vi "Cartesian To Complex - R,RM.vi"(1 "Real Matrix I":T1, 2 "Real Scalar r":dbl) -> (0 "r + Ii":T2)   [LabVIEW 2017, in "NI_Matrix.lvlib"]
doc: "Creates a complex number from two values in rectangular notation."
uses:
  NI_Matrix.lvlib
  ComplexMatrix.ctl
  RealMatrix.ctl
  Array To Matrix - CA2.vi
  Matrix To Array - RM.vi
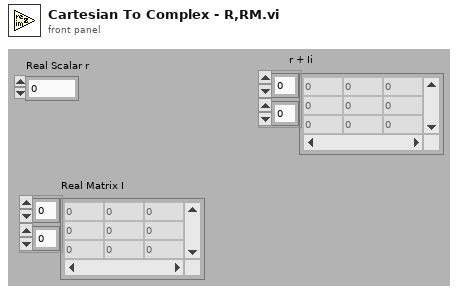
[diagram p1: front panel]
types:
  T1 = typedef "NI_Matrix.lvlib/RealMatrix.ctl" = dbl[][]
  T2 = typedef "NI_Matrix.lvlib/ComplexMatrix.ctl" = cdb[][]
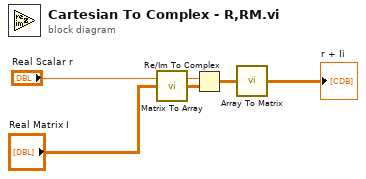
[diagram p0: block diagram]
diagram:
  n1 = call-poly "Matrix To Array.vi"("Real Matrix"="Real Matrix I") -> ("Real 2D Array"=w4:dbl[][])
  n2 = Re/Im To Complex(1:w4, 2:"Real Scalar r") -> (0:w2:cdb[][])
  n3 = call-poly "Array To Matrix.vi"("Complex 2D Array"=w2) -> ("Complex Matrix"=→"r + Ii":T2)
